vi "Read Default channels.vi"(8 "error in (no error)":errorcluster, 11 "Common Measurements in":refnum<class "Common Measurements.lvclass">) -> (0 "error out":errorcluster, 1 "Keep old\nplots":bool, 2 "Default channels":string[][](array[string]), 3 "Common Measurements out":refnum<class "Common Measurements.lvclass">)   [LabVIEW 2015, in "Common Measurements.lvclass"]
uses:
  Common Measurements.lvclass
  Common Measurements.lvclass/Common Measurements.ctl
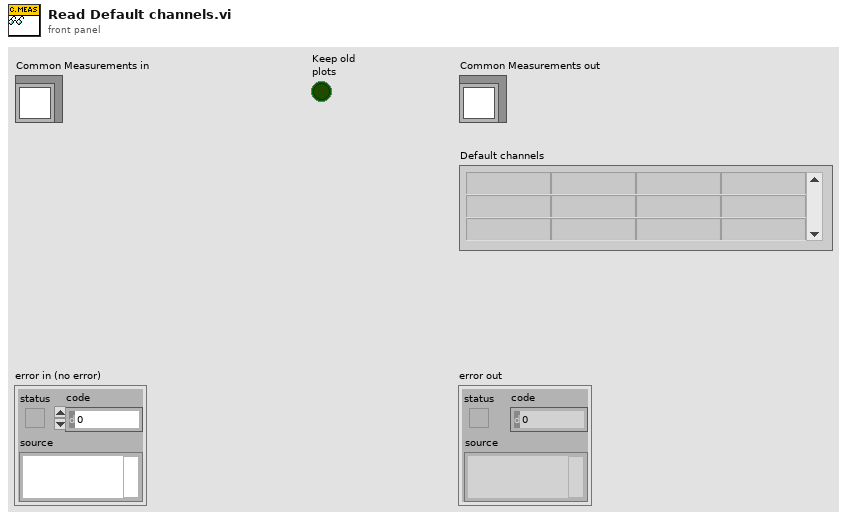
[diagram p1: front panel]
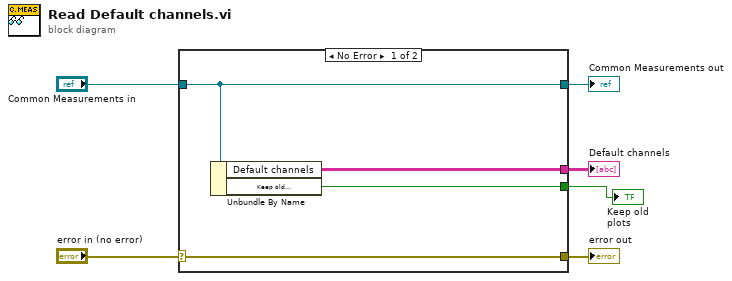
[diagram p0: block diagram]
diagram:
  n1 = case shown="No Error" "error in (no error)" {
    selector: "error in (no error)" -> [w10 w11]
    tunnel: [w10 w11] -> w5
    tunnel: [w9 w12] -> w3
    tunnel: "Common Measurements in" -> [w9 w12]
    tunnel: [w8 _] -> w2
    tunnel: [w7 _] -> w1
    frame No Error {
      n2 = Unbundle By Name(w9) -> ("Default channels"=w8:string[][], "Keep old\nplots"=w7:bool)
    }
    frame Error {
    }
  }
  "error out" <- w5
  "Common Measurements out" <- w3
  "Default channels" <- w2
  "Keep old\nplots" <- w1
